vi "Read All Datatype Information.vi"(8 "error in (no error)":errorcluster, 11 "TwinCAT ADS in":refnum<class "TwinCAT ADS.lvclass">) -> (0 "error out":errorcluster, 1 "Data Type Information":T1[](array[typedef]) {"Category" items=["Unknown, None"=0, "Primitive"=1, "Alias"=2, "Enum"=3, "Array"=4, "Struct"=5, "FunctionBlock"=6, "Program"=7, "Function"=8, "SubRange"=9, "String"=10, "Bitset"=12, "Pointer"=13, "Union"=14, "Reference"=15, "Interface"=16]; "Type ID" items=["ADST_VOID"=0, "ADST_INT16"=2, "ADST_INT32"=3, "ADST_REAL32"=4, "ADST_REAL64"=5, "ADST_INT8"=16, "ADST_UINT8"=17, "ADST_UINT16"=18, "ADST_UINT32"=19, "ADST_INT64"=20, "ADST_UINT64"=21, "ADST_STRING"=30, "ADST_WSTRING"=31, "ADST_REAL80"=32, "ADST_BIT"=33, "ADST_MAXTYPES"=34, "ADST_BIGTYPE"=65]}, 3 "TwinCAT ADS out":refnum<class "TwinCAT ADS.lvclass">)   [LabVIEW 2018, in "TwinCAT ADS.lvclass"]
uses:
  TwinCAT ADS.lvclass
  Controls/Datatype Information.ctl
  TwinCAT ADS.lvclass/TwinCAT ADS.ctl
  Get Type Map.vi
  TwinCAT.Ads
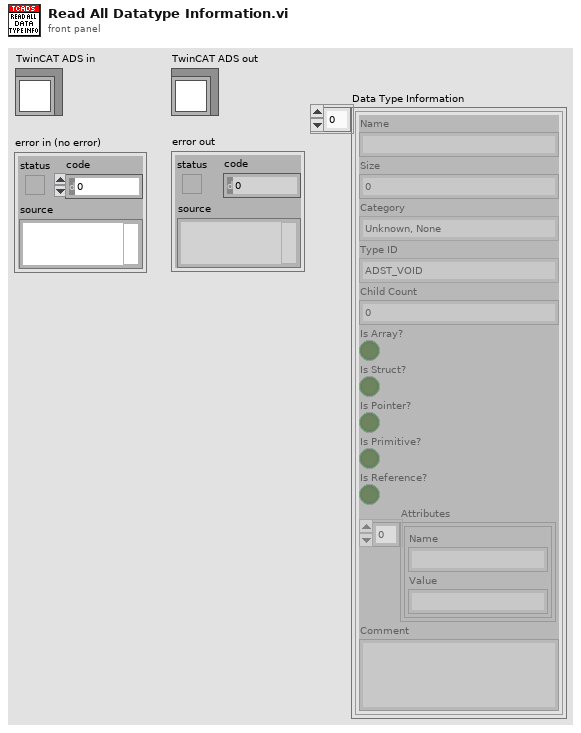
[diagram p1: front panel]
types:
  T1 = typedef "TwinCAT ADS.lvclass/Datatype Information.ctl" = cluster{"Name":string, "Size":i32, "Category":i32, "Type ID":i32, "Child Count":i32, "Is Array?":bool, "Is Struct?":bool, "Is Pointer?":bool, "Is Primitive?":bool, "Is Reference?":bool, "Attributes":cluster{"Name":string, "Value":string}[], "Comment":string}
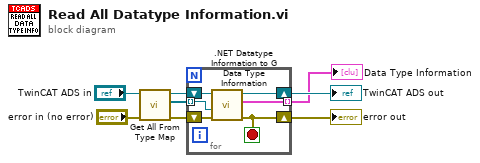
[diagram p0: block diagram]
diagram:
  n1 = call "Get All From Type Map.vi"("error in (no error)"="error in (no error)", "TwinCAT ADS in"="TwinCAT ADS in") -> ("error out"=w4:errorcluster, "[.NET AdsDataType]"=w2:refnum<k24>[], "TwinCAT ADS out"=w3:refnum<class "TwinCAT ADS.lvclass">)  [unwired: 7 in]
  n2 = for {
    shift-right: [w12] -> w8
    shift-left: w4 -> [w9]
    tunnel: [w11] -> w5 mode=indexing
    tunnel: w2 -> [w10] mode=indexing
    shift-right: [w13] -> w6
    shift-left: w3 -> [w14]
    stop <- w12 stop-if-true
    n3 = call ".NET Datatype Information to G Data Type Information.vi"("error in (no error)"=w9, ".NET Data Type Information"=w10, "TwinCAT ADS in"=w14) -> ("error out"=w12:errorcluster, "Data Type Information"=w11:T1, "TwinCAT ADS out"=w13:refnum<class "TwinCAT ADS.lvclass">)  [unwired: 6 in]
  }
  "error out" <- w8
  "TwinCAT ADS out" <- w6
  "Data Type Information" <- w5
